vi "RunProbeCycle.vi"(10 "UiDefinition":T1) -> ()   [LabVIEW 2020]
uses:
  UIReferences.ctl
  C:/Users/User/Desktop/Automation/CurrentVersion/LabviewDXFViewer/bin/Release/LabviewDXFViewer.exe
  LabviewDXFViewer/bin/Release/LabviewDXFViewer.exe
  <vilib>/Utility/file.llb/Write Delimited Spreadsheet (string).vi
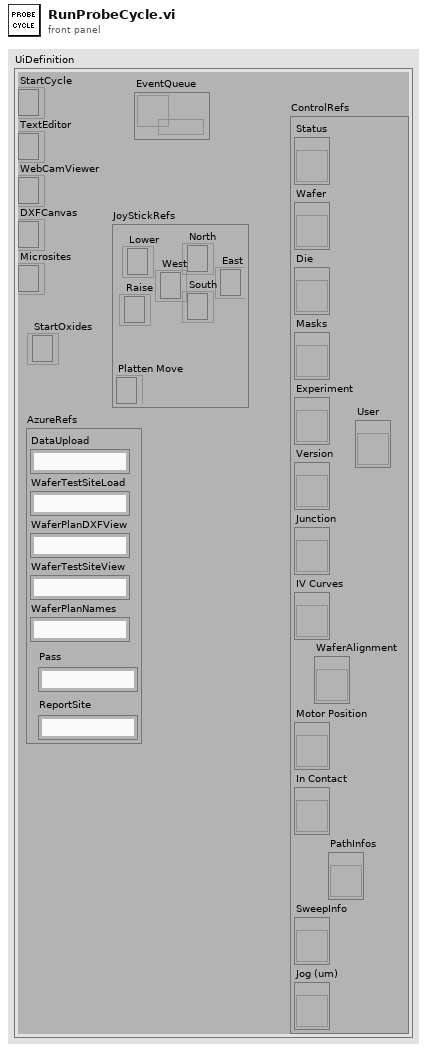
[diagram p1: front panel]
types:
  T1 = typedef "UIReferences.ctl" = cluster{"StartCycle":refnum<k24>, "TextEditor":refnum<k24>, "WebCamViewer":refnum<k24>, "DXFCanvas":refnum<k24>, "Microsites":refnum<k24>, "JoyStickRefs":cluster{"North":refnum<k24>, "Lower":refnum<k24>, "Raise":refnum<k24>, "Platten Move":refnum<k24>, "West":refnum<k24>, "East":refnum<k24>, "South":refnum<k24>}, "AzureRefs":cluster{"DataUpload":string, "WaferTestSiteLoad":string, "WaferPlanDXFView":string, "WaferTestSiteView":string, "WaferPlanNames":string, "Pass":string, "ReportSite":string}, "ControlRefs":cluster{"Status":refnum<vi>, "Wafer":refnum<vi>, "Die":refnum<vi>, "Masks":refnum<vi>, "Experiment":refnum<vi>, "Version":refnum<vi>, "Junction":refnum<vi>, "IV Curves":refnum<vi>, "Motor Position":refnum<vi>, "In Contact":refnum<vi>, "SweepInfo":refnum<vi>, "Jog (um)":refnum<vi>, "PathInfos":refnum<vi>, "User":refnum<vi>, "WaferAlignment":refnum<vi>}, "EventQueue":refnum<queue>, "StartOxides":refnum<k24>}
  T2 = cluster{"Current Range":dbl, "Source Measure Unit Channel (0: Channel A)":i32, "Waveform":waveform(dbl), "VISA resource name":refnum<visa-resource-name>, "CodeText":string}
  T3 = cluster{"Die":string, "Wafer":string, "Path":path, "url":string, "Experiment":string, "Version":string, "user":string}
  T4 = typedef "WaferAlignmentType.ctl" = cluster{"Wafer Units to microns":dbl, "Rotation Misalign":dbl[], "Scale Misalign":dbl, "Steps Per micron":dbl, "Position 1":i32[], "Position 2":i32[], "Lift Distance":i32, "Position 3":i32[], "Jog Height":i32}
  T5 = cluster{"Coordinates":dbl[], "Junction Name":string, "Orientation":string}[]
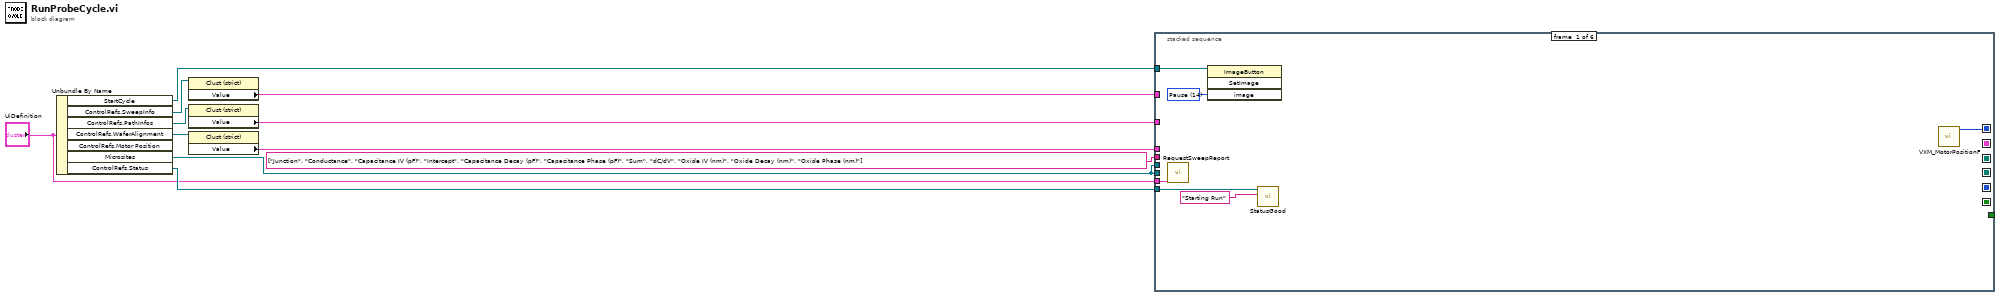
[diagram p0: block diagram]
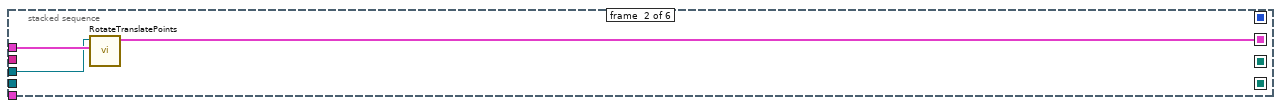
[diagram p2: hidden frame]
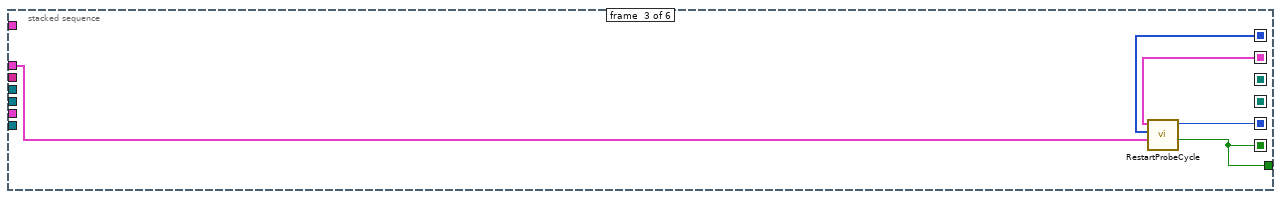
[diagram p3: hidden frame]
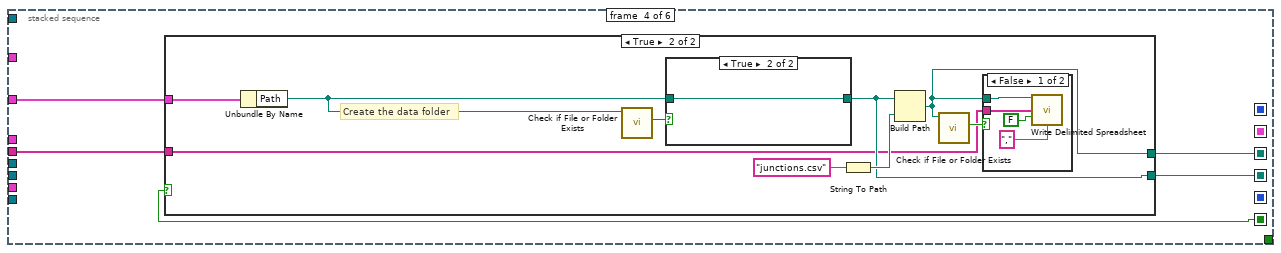
[diagram p4: hidden frame]
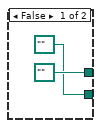
[diagram p5: hidden frame]
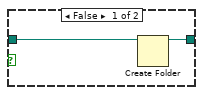
[diagram p7: hidden frame]
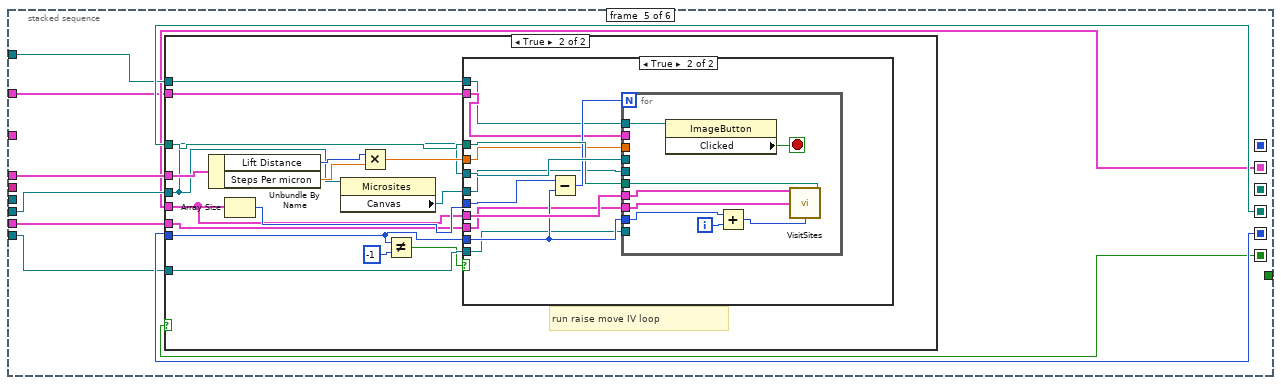
[diagram p8: hidden frame]
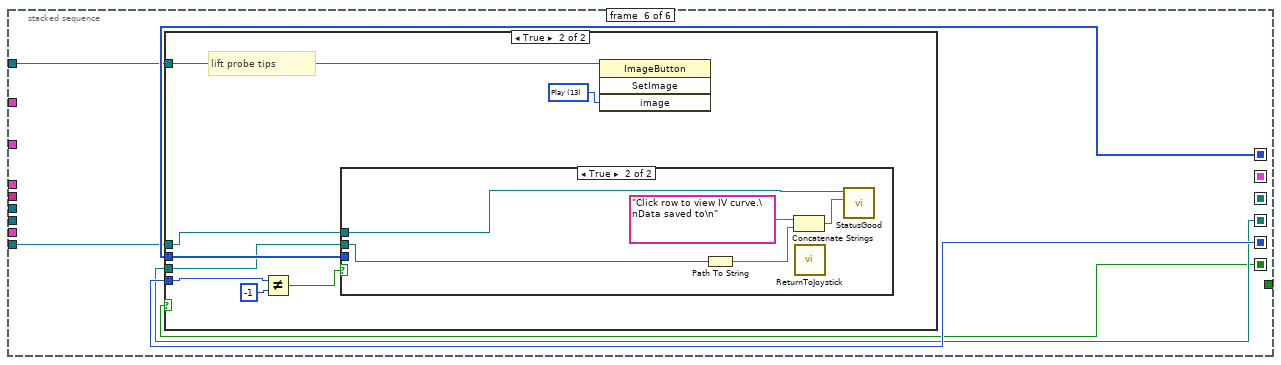
[diagram p11: hidden frame]
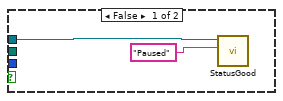
[diagram p13: hidden frame]
diagram:
  n1 = Unbundle By Name("UiDefinition") -> ("StartCycle"=w11:refnum<k24>, "ControlRefs.SweepInfo"=w10:refnum<vi>, "ControlRefs.PathInfos"=w7:refnum<vi>, "ControlRefs.WaferAlignment"=w6:refnum<vi>, "Microsites"=w3:refnum<k24>, "ControlRefs.Status"=w5:refnum<vi>)  [unwired: 1 out]
  n2 = property class="Clust (strict)"(reference=w10) -> ("Value"=w9:T2)  [unwired: 1 in, 2 out]
  n3 = property class="Clust (strict)"(reference=w7) -> ("Value"=w8:T3)  [unwired: 1 in, 2 out]
  n4 = property class="Clust (strict)"(reference=w6) -> ("Value"=w4:T4)  [unwired: 1 in, 2 out]
  n5 = stacked-sequence {
    seq-local: [_ w20 _ _ _ _] -> [_ _ w22 _ w52 _]
    seq-local: [w17 _ _ _ _ _] -> [_ _ w24 _ _ w100]
    seq-local: [_ _ _ w29 _ _] -> [_ _ _ _ w58 w97]
    seq-local: [_ _ w25 _ _ _] -> [_ _ _ _ w57 w99]
    seq-local: [_ _ _ w28 _ _] -> [_ _ _ _ _ _]
    seq-local: [_ _ w21 _ _ _] -> [_ _ _ w26 w49 w95]
    tunnel: w3 -> [_ _ _ _ w53 _]
    tunnel: w8 -> [_ _ _ w30 _ _]
    tunnel: w9 -> [_ _ _ _ w50 _]
    tunnel: w11 -> [w16 _ _ _ w56 w98]
    tunnel: w5 -> [w13 _ _ _ w55 w96]
    tunnel: w4 -> [_ w19 w23 _ w54 _]
    tunnel: w3 -> [_ w18 _ _ _ _]
    tunnel: "UiDefinition" -> [w12 _ _ _ w51 _]
    tunnel: string[] ["Junction", "Conductance", "Capacitance IV (pF)", "Intercept", "Capacitance Decay (pF)", "Capacitance Phase (pF)", "Sum", "dC/dV", "Oxide IV (nm)", "Oxide Decay (nm)", "Oxide Phase (nm)"] -> [_ _ _ w27 _ _]
    tunnel: [_ _ w21 _ _ _] -> _
    frame #0 {
      w15 = 14 items=["Left", "LeftBig", "LeftSmall", "Right", "RightBig", "RightSmall", "Up", "UpBig", "UpSmall", "Down", "DownBig", "DownSmall", "Zero", "Play", "Pause", "Load", "Lower", "Raise", "Home", "Home2"] ("image")
      n6 = call "RequestSweepReport.vi"("UiDefinition 2"=w12) -> ()  [unwired: 11 in]
      n7 = invoke class="ImageButton" method="SetImage"(reference=w16, "image"=w15) -> ()  [unwired: 2 in, 4 out]
      n8 = call "StatusGood.vi"("Text.Text"="Starting Run" ("Run Message"), "String in"=w13) -> ()  [unwired: 10 in]
      n9 = call "VXM_MotorPositionF.vi"() -> ("Position"=w17:i32[])  [unwired: 11 in]
    }
    frame #1 {
      n10 = call "RotateTranslatePoints.vi"("WaferAlignment"=w19, ".NET Refnum in"=w18) -> ("Array"=w20:T5)  [unwired: 9 in]
    }
    frame #2 {
      n11 = call "RestartProbeCycle.vi"("WaferAlignment"=w23, "Position"=w24, "Array"=w22) -> ("In Starting Position"=w21:bool, "Numeric"=w25:i32)  [unwired: 7 in]
    }
    frame #3 {
      n12 = case shown="True" w26 {
        tunnel: w30 -> [_ w38]
        tunnel: [path "" ("Path") w37] -> w29
        tunnel: [path "" ("appended path") w34] -> w28
        tunnel: w27 -> [_ w33]
        frame False {
        }
        frame True {
          # "Create the data folder"
          n13 = Unbundle By Name(w38) -> ("Path"=w36:path)
          n14 = call <vilib>:"Check if File or Folder Exists.vi"("path"=w36) -> ("file or folder exists?"=w41:bool)  [unwired: 8 in, 2 out]
          n15 = case shown="True" w41 {
            tunnel: w36 -> [w47 w48]
            tunnel: [w46 w48] -> w37
            frame False {
              n16 = Create Folder(path (use dialog)=w47) -> (created path=w46:path)  [unwired: 2 in, 2 out]
            }
            frame True {
            }
          }
          n17 = String To Path(string="junctions.csv") -> (path=w40:path)
          n18 = Build Path(base path=w37, name or relative path=w40) -> (appended path=w34:path)
          n19 = call <vilib>:"Check if File or Folder Exists.vi"("path"=w34) -> ("file or folder exists?"=w35:bool)  [unwired: 8 in, 2 out]
          n20 = case shown="False" w35 {
            tunnel: w34 -> [w45 _]
            tunnel: w33 -> [w42 _]
            frame False {
              n21 = call-poly <vilib>:"Write Delimited Spreadsheet.vi"("file path (dialog if empty)"=w45, "1D data"=w42, "append to file? (new file:F)"=FALSE, "delimiter (\\t)"="," ("delimiter (\\t)")) -> ()  [unwired: 10 in, 2 out]
            }
            frame True {
            }
          }
        }
      }
    }
    frame #4 {
      n22 = case shown="True" w49 {
        tunnel: w58 -> [_ w74]
        tunnel: w57 -> [_ w72]
        tunnel: w56 -> [_ w70]
        tunnel: w55 -> [_ w69]
        tunnel: w54 -> [_ w68]
        tunnel: w53 -> [_ w63]
        tunnel: w52 -> [_ w62]
        tunnel: w51 -> [_ w61]
        tunnel: w50 -> [_ w60]
        frame False {
        }
        frame True {
          # "run raise move IV loop"
          n23 = Unbundle By Name(w68) -> ("Lift Distance"=w67:i32, "Steps Per micron"=w66:dbl)
          n24 = Array Size(array=w62) -> (size(s)=w73:i32)
          n25 = property class="Microsites"(reference=w63) -> ("Canvas"=w64:refnum<k24>)  [unwired: 1 in, 2 out]
          n26 = Multiply(x=w67, y=w66) -> (x*y=w65:dbl)
          n27 = Not Equal?(x=w72, y=-1) -> (x != y?=w59:bool)
          n28 = case shown="True" w59 {
            tunnel: w62 -> [_ w86]
            tunnel: w63 -> [_ w85]
            tunnel: w74 -> [_ w84]
            tunnel: w72 -> [_ w81]
            tunnel: w73 -> [_ w82]
            tunnel: w60 -> [_ w80]
            tunnel: w70 -> [_ w79]
            tunnel: w69 -> [_ w78]
            tunnel: w65 -> [_ w77]
            tunnel: w64 -> [_ w76]
            tunnel: w61 -> [_ w75]
            frame False {
            }
            frame True {
              n29 = Subtract(x=w82, y=w81) -> (x-y=w83:i32)
              n30 = for {
                N: w83 -> [_]
                tunnel: w77 -> [_]
                tunnel: w86 -> [w91]
                tunnel: w85 -> [_]
                tunnel: w84 -> [w92]
                tunnel: w81 -> [w93]
                tunnel: w80 -> [_]
                tunnel: w79 -> [w89]
                tunnel: w78 -> [_]
                tunnel: w76 -> [_]
                tunnel: w75 -> [w90]
                i -> [w94]
                stop <- w88 stop-if-true
                n31 = property class="ImageButton"(reference=w89) -> ("Clicked"=w88:bool)  [unwired: 1 in, 2 out]
                n32 = Add(x=w93, y=w94) -> (x+y=w87:i32)
                n33 = call "VisitSites.vi"("Microsites"=w91, "Path"=w92, "UiDefinition"=w90, "CurrentPositionIndex"=w87) -> ()  [unwired: 12 in]
              }
            }
          }
        }
      }
    }
    frame #5 {
      n34 = case shown="True" w95 {
        tunnel: w100 -> [_ w108]
        tunnel: w99 -> [_ w106]
        tunnel: w98 -> [_ w104]
        tunnel: w97 -> [_ w102]
        tunnel: w96 -> [_ w101]
        frame False {
        }
        frame True {
          w103 = 13 items=["Left", "LeftBig", "LeftSmall", "Right", "RightBig", "RightSmall", "Up", "UpBig", "UpSmall", "Down", "DownBig", "DownSmall", "Zero", "Play", "Pause", "Load", "Lower", "Raise", "Home", "Home2"] ("image")
          # "lift probe tips"
          n35 = Not Equal?(x=w106, y=-1) -> (x != y?=w105:bool)
          n36 = case shown="True" w105 {
            tunnel: w108 -> [_ _]
            tunnel: w102 -> [_ w115]
            tunnel: w101 -> [w110 w114]
            frame False {
              n37 = call "StatusGood.vi"("Text.Text"="Paused", "String in"=w110) -> ()  [unwired: 10 in]
            }
            frame True {
              n38 = Path To String(path=w115) -> (string=w113:string)
              n39 = Concatenate Strings("Click row to view IV curve.\nData saved to\n" ("Text.Text"), w113) -> (w111:string)
              n40 = call "ReturnToJoystick.vi"() -> ()  [unwired: 12 in]
              n41 = call "StatusGood.vi"("Text.Text"=w111, "String in"=w114) -> ()  [unwired: 10 in]
            }
          }
          n42 = invoke class="ImageButton" method="SetImage"(reference=w104, "image"=w103) -> ()  [unwired: 2 in, 4 out]
        }
      }
    }
  }
